vi "Update Config.vi"(8 "error in (no error)":errorcluster, 11 "SignalConfig":T1={"VPP"=0, "Frecuency"=50.0, "Offset"=0.0, "signal type"=enum."Sine Wave"}) -> (0 "error out":errorcluster)   [LabVIEW 2020, in "DataBase.lvlib"]
uses:
  DataBase.lvlib
  Acquisition/SignalConfig--cluster.ctl
  <vilib>/drjdpowell/SQLite Library/SQL Connection/Open (path).vi
  <vilib>/drjdpowell/SQLite Library/SQL Connection/Open (string).vi
  <vilib>/AdvancedString/Path To Command Line String.vi
  <vilib>/drjdpowell/SQLite Library/SQL Connection/Execute SQL (No results).vi
  <vilib>/drjdpowell/SQLite Library/SQL Connection/Connection.lvclass
  <vilib>/drjdpowell/SQLite Library/SQLite.lvlib
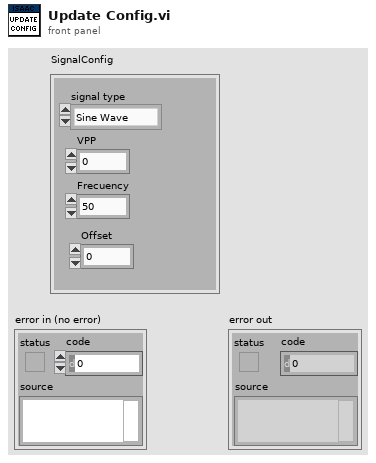
[diagram p1: front panel]
types:
  T1 = typedef "SignalConfig--cluster.ctl" = cluster{"VPP":i32, "Frecuency":dbl, "Offset":dbl, "signal type":enum16{"Sine Wave", "Triangle Wave", "Square Wave", "Sawtooth Wave"}}
  T2 = enum16{"Sine Wave", "Triangle Wave", "Square Wave", "Sawtooth Wave"}
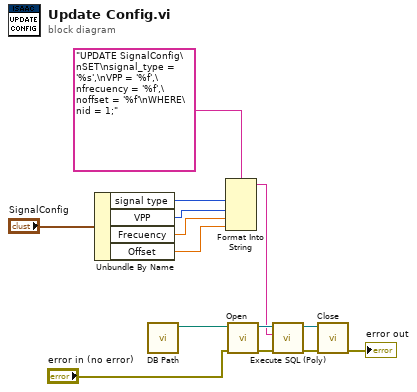
[diagram p0: block diagram]
diagram:
  n1 = Unbundle By Name("SignalConfig") -> ("signal type"=w4:T2, "VPP"=w3:i32, "Frecuency"=w2:dbl, "Offset"=w1:dbl)
  n2 = call "DB Path.vi"() -> ("appended path"=w8:path)  [unwired: 11 in]
  n3 = Format Into String(format string="UPDATE SignalConfig\nSET\nsignal_type = '%s',\nVPP = '%f',\nfrecuency = '%f',\noffset = '%f'\nWHERE\nid = 1;", w4, w3, w2, w1) -> (resulting string=w10:string)  [unwired: 2 in, 1 out]
  n4 = call-poly <vilib>:"Open.vi"("error in (no error)"="error in (no error)", "db file"=w8) -> ("error out"=w14:errorcluster, "SQLite Connection"=w13:refnum<class "Connection.lvclass">)  [unwired: 8 in]
  n5 = call-poly <vilib>:"Execute SQL (Poly).vi"("error in (no error)"=w14, "SQL"=w10, "SQLite Connection in"=w13) -> ("error out"=w12:errorcluster, "SQLite Connection"=w11:refnum<class "Connection.lvclass">)  [unwired: 7 in]
  n6 = call-dynamic "Close.vi"("error in (no error)"=w12, "SQLite Connection in"=w11) -> ("error out"=→"error out":errorcluster)  [unwired: 9 in]
